vi "AssertValueByFocusName.vi"(0 "VI Reference In":refnum<vi>, 1 "Test Label":string, 2 "delimiter (>>)":string=">>", 3 "Assert Only? (F)":bool, 5 "Control Path":string, 7 "Item Name":string, 11 "Error In":errorcluster, 12 "Assert Interval(10 ms)":u32=10, 13 "Timeout(5 sec)":dbl=5.0) -> (4 "VI Reference Out":refnum<vi>, 6 "Asserted Value":string, 15 "Error Out":errorcluster)   [LabVIEW 2016, in "Drona.lvlib" / "AssertControlValue.lvlib" / "AssertListbox.lvlib"]
doc: "Asserts if the focus item name on listbox controls is equal.\n\nThe input control name is given as a string , incase of path, use delimiters inbetween the path.\nThis VI gets the value of the control, untill the value is equal to the input value."
uses:
  AssertListbox.lvlib
  Get/GetControlRef/GetControlRefByPath.vi
  <vilib>/addons/_JKI Toolkits/Caraya/classes/Assert/Assert Equal Value_Variant.vi
  <vilib>/addons/_JKI Toolkits/Caraya/classes/Assert/Assert.lvclass
  Get/GetControlRef/GetControlRef.lvlib
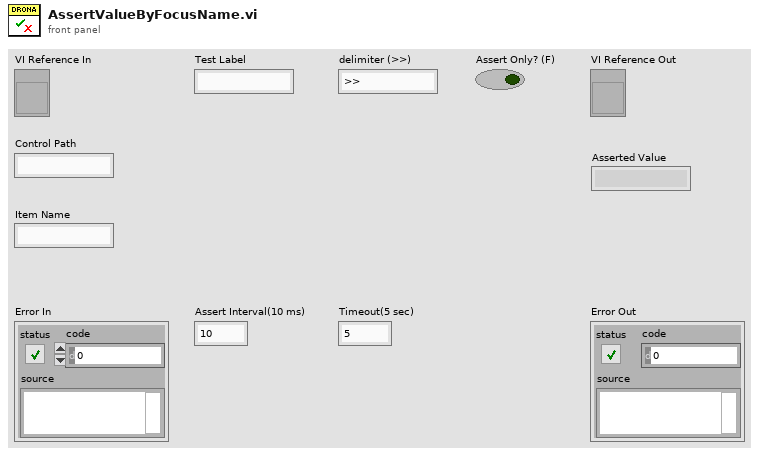
[diagram p1: front panel]
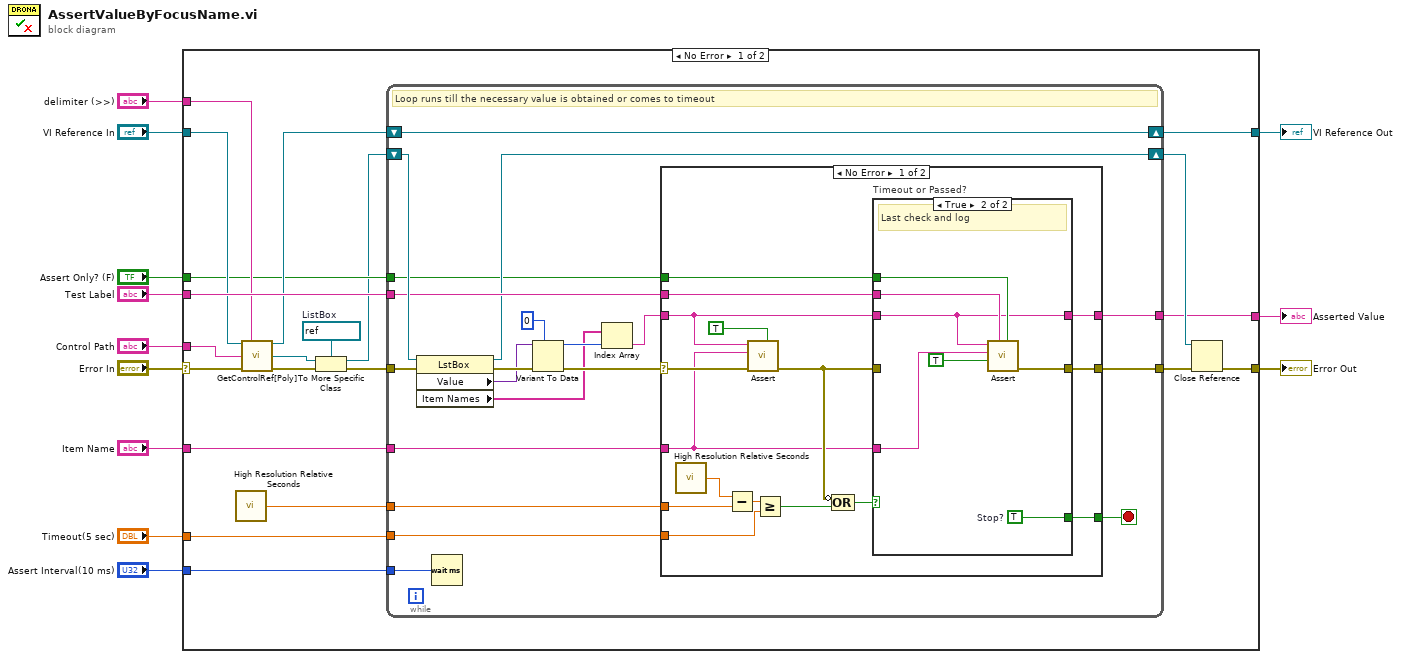
[diagram p0: block diagram]
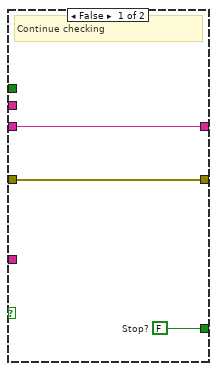
[diagram p2: hidden frame]
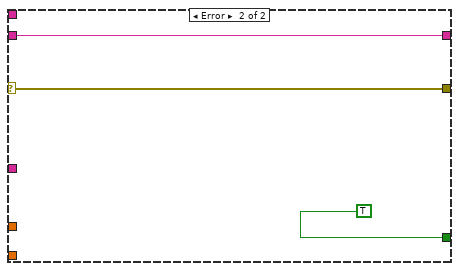
[diagram p3: hidden frame]
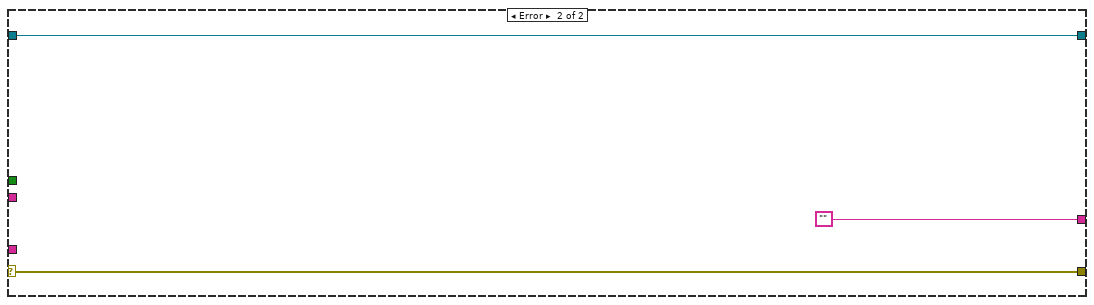
[diagram p4: hidden frame]
diagram:
  n1 = case shown="No Error" "Error In" {
    selector: "Error In" -> [w27 w85]
    tunnel: "Timeout(5 sec)" -> [w33 _]
    tunnel: [w32 w84] -> w11
    tunnel: "Item Name" -> [w31 _]
    tunnel: [w21 w85] -> w10
    tunnel: "Assert Interval(10 ms)" -> [w29 _]
    tunnel: "Test Label" -> [w28 _]
    tunnel: "VI Reference In" -> [w26 w84]
    tunnel: "Control Path" -> [w25 _]
    tunnel: "delimiter (>>)" -> [w19 _]
    tunnel: "Assert Only? (F)" -> [w18 _]
    tunnel: [w17 ""] -> w1
    frame No Error {
      w14 = refnum<vi> refnum  # ListBox
      n2 = call <vilib>:"High Resolution Relative Seconds.vi"() -> ("relative seconds"=w24:dbl)
      n3 = call-poly "GetControlRef[Poly].vi"("VI Reference In"=w26, "delimiter (>>)"=w19, "Control Path"=w25, "error In"=w27) -> ("VI Reference Out"=w22:refnum<vi>, "Ctl Refnum"=w15:refnum<vi>, "error out"=w23:errorcluster)  [unwired: 9 in]
      n4 = To More Specific Class(target class=w14, reference=w15, error in=w23) -> (specific class reference=w13:refnum<vi>, error out=w16:errorcluster)
      n5 = while {
        tunnel: w31 -> [w40]
        tunnel: w33 -> [w52]
        tunnel: w24 -> [w53]
        tunnel: w16 -> [w47]
        tunnel: [w50] -> w30
        tunnel: w29 -> [w48]
        tunnel: w28 -> [w44]
        shift-right: [w45] -> w32
        shift-left: w22 -> [w45]
        shift-right: [w43] -> w20
        shift-left: w13 -> [w46]
        tunnel: w18 -> [w42]
        tunnel: [w41] -> w17
        stop <- w51 stop-if-true
        # "Loop runs till the necessary value is obtained or comes to timeout"
        n6 = property on="Property Node" class="LstBox"(reference=w46, error in=w47) -> (reference out=w43:refnum<vi>, error out=w49:errorcluster, "Value"=w38:variant, "Item Names"=w34:string[])
        n7 = Wait (ms)(milliseconds to wait=w48) -> ()  [unwired: 1 out]
        n8 = Variant To Data(error in=w49, type=0, Variant=w38) -> (data=w36:i32, error out=w39:errorcluster)
        n9 = Index Array(array=w34, index=w36) -> (element=w35:string)
        n10 = case shown="No Error" w39 {
          selector: w39 -> [w65 w82]
          tunnel: w53 -> [w69 _]
          tunnel: w52 -> [w66 _]
          tunnel: [w56 TRUE] -> w51
          tunnel: [w57 w82] -> w50
          tunnel: w40 -> [w58 _]
          tunnel: w35 -> [w59 w80]
          tunnel: w44 -> [w64 _]
          tunnel: w42 -> [w55 _]
          tunnel: [w54 w80] -> w41
          frame No Error {
            n11 = call <vilib>:"High Resolution Relative Seconds.vi"() -> ("relative seconds"=w68:dbl)
            n12 = Subtract(x=w68, y=w69) -> (x-y=w67:dbl)
            n13 = call-poly <vilib>:"Assert.vi"("Assert Only? (F)"=TRUE, "error in (no error)"=w65, "Y"=w58, "X"=w59) -> ("error out"=w62:errorcluster)  [unwired: 7 in]
            n14 = Greater Or Equal?(x=w67, y=w66) -> (x >= y?=w63:bool)
            n15 = Compound Arithmetic op=OR(invert w62, w63) -> (w61:bool)
            n16 = case "Timeout or Passed?" shown="True" w61 {
              tunnel: w62 -> [w72 _]
              tunnel: w58 -> [_ w75]
              tunnel: w59 -> [w70 w74]
              tunnel: w64 -> [_ w79]
              tunnel: [w72 w78] -> w57
              tunnel: [w71 w77] -> w56
              tunnel: w55 -> [_ w76]
              tunnel: [w70 w74] -> w54
              frame False {
                w71 = FALSE  # Stop?
                # "Continue checking"
              }
              frame True {
                w77 = TRUE  # Stop?
                # "Last check and log"
                n17 = call-poly <vilib>:"Assert.vi"("Assert Only? (F)"=w76, "Label"=w79, "Register with caller test (F)"=TRUE, "Y"=w75, "X"=w74) -> ("error out"=w78:errorcluster)  [unwired: 6 in]
              }
            }
          }
          frame Error {
          }
        }
      }
      n18 = Close Reference(reference=w20, error in (no error)=w30) -> (error out=w21:errorcluster)
    }
    frame Error {
    }
  }
  "Error Out" <- w10
  "VI Reference Out" <- w11
  "Asserted Value" <- w1
